vi "ManualLauncher.vi"() -> ()   [LabVIEW 2012]
uses:
  LauncherPresets.ctl
  Sally_Dashboard_2013/DBNameEnum.ctl
  Robot Global Data.vi
panel:
  in  "LauncherPresets":T1
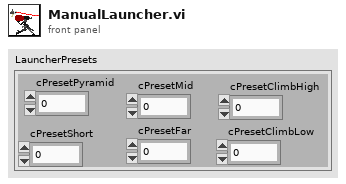
[diagram p1: front panel]
types:
  T1 = typedef "LauncherPresets.ctl" = cluster{"cPresetPyramid":dbl, "cPresetShort":dbl, "cPresetMid":dbl, "cPresetFar":dbl, "cPresetClimbHigh":dbl, "cPresetClimbLow":dbl}
  T2 = typedef "DBNameEnum.ctl" = enum16{"AutoInstructions", "DriveLoopTime", "DriveAlignLSLeft", "DriveAlignLSRight", "Use2DriveAlign", "ClimbLS", "LauncherAngleMatches", "FrameworkVersion", "sLauncherAngle", "LauncherTargetAngle", "sLauncherRPM", "LauncherTargetRPM", "sDriveDistance", "LauncherMotorValue", "PullbackTol", "FireTol", "LauncherRPMTol", "LauncherAngleTol", "InitialWait", "WaitBetweenLaunch", "AnglePresets", "RPMPresets", "UseAngleEncoder", "UseLauncherEncoder", "UseLauncherPID", "QSWaitBeforeFire", "QSWaitBeforeRetract", "AngleForwardValue", "AngleBackwardValue", "UseClusterArray", "BackupAuto", "ReverseDriveIndicate", "HalfSpeedFactor"}
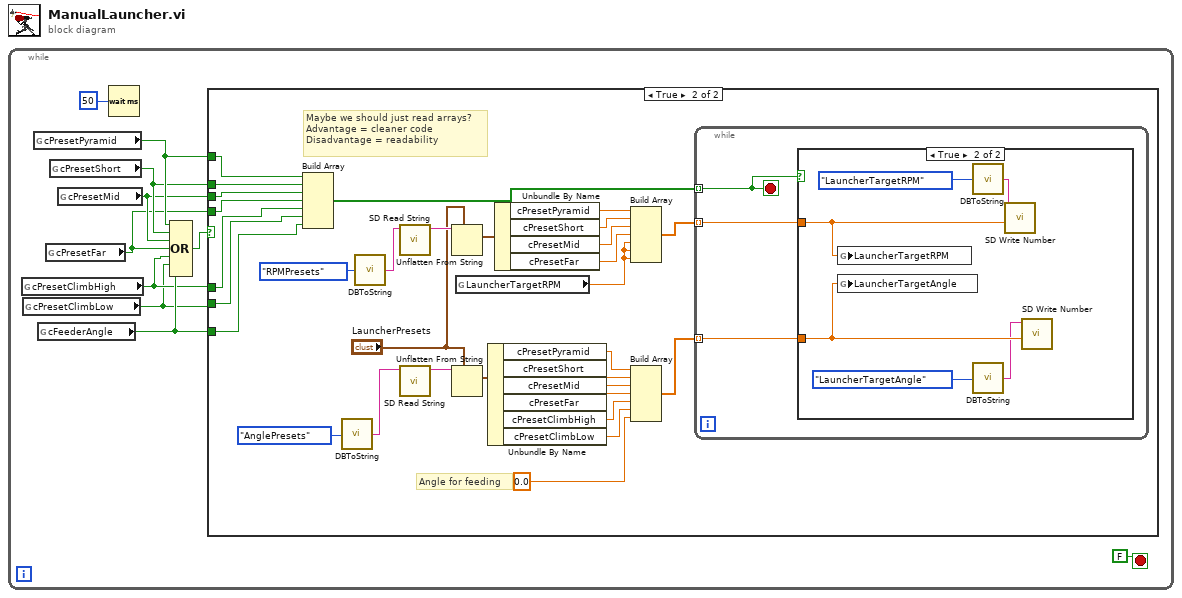
[diagram p0: block diagram]
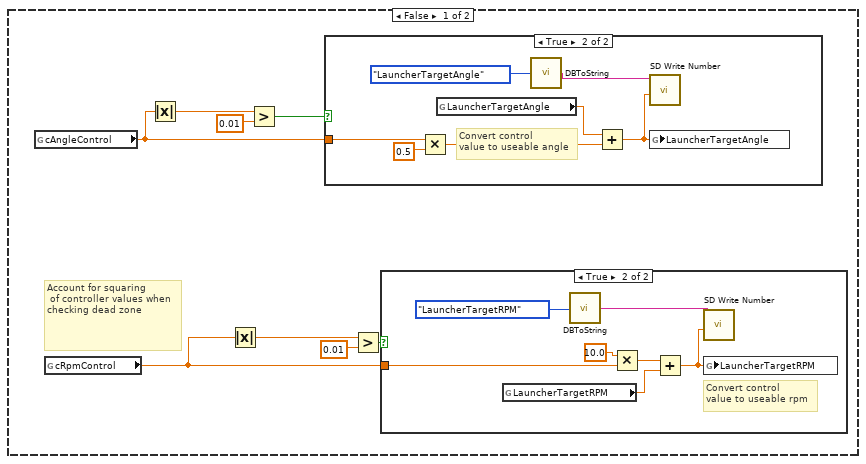
[diagram p2: hidden frame]
diagram:
  n1 = while {
    stop <- FALSE stop-if-true
    n2 = global read "Robot Global Data.vi" "cPresetClimbHigh"() -> (w2:bool)
    n3 = global read "Robot Global Data.vi" "cPresetClimbLow"() -> (w1:bool)
    n4 = global read "Robot Global Data.vi" "cPresetPyramid"() -> (w8:bool)
    n5 = global read "Robot Global Data.vi" "cFeederAngle"() -> (w3:bool)
    n6 = global read "Robot Global Data.vi" "cPresetFar"() -> (w5:bool)
    n7 = global read "Robot Global Data.vi" "cPresetShort"() -> (w7:bool)
    n8 = global read "Robot Global Data.vi" "cPresetMid"() -> (w6:bool)
    n9 = Wait (ms)(milliseconds to wait=u32 50) -> ()  [unwired: 1 out]
    n10 = Compound Arithmetic op=OR(w8, w7, w6, w5, w2, w1, w3) -> (w9:bool)
    n11 = case shown="True" w9 {
      tunnel: w8 -> [_ w63]
      tunnel: w7 -> [_ w62]
      tunnel: w6 -> [_ w61]
      tunnel: w5 -> [_ w60]
      tunnel: w3 -> [_ w33]
      tunnel: w2 -> [_ w35]
      tunnel: w1 -> [_ w34]
      frame False {
        # "Account for squaring\n of controller values when checking dead zone"
        n12 = global read "Robot Global Data.vi" "cAngleControl"() -> (w14:dbl)
        n13 = global read "Robot Global Data.vi" "cRpmControl"() -> (w16:dbl)
        n14 = Absolute Value(x=w14) -> (abs(x)=w15:dbl)
        n15 = Absolute Value(x=w16) -> (abs(x)=w17:dbl)
        n16 = Greater?(x=w15, y=0.01) -> (0:w13:bool)
        n17 = case shown="True" w13 {
          tunnel: w14 -> [_ w25]
          frame False {
          }
          frame True {
            # "Convert control\nvalue to useable angle"
            n18 = Multiply(x=w25, y=0.5) -> (x*y=w22:dbl)
            n19 = global read "Robot Global Data.vi" "LauncherTargetAngle"() -> (w23:dbl)
            n20 = call "DBToString.vi"("Enum"=DBNameEnum."LauncherTargetAngle") -> ("Refname"=w19:string)
            n21 = Add(x=w23, y=w22) -> (x+y=w21:dbl)
            n22 = call <vilib>:"SD Write Number.vi"("Numeric"=w21, "Name"=w19) -> ()  [unwired: 8 in, 2 out]
            n23 = global write "Robot Global Data.vi" "LauncherTargetAngle"(w21) -> ()
          }
        }
        n24 = Greater?(x=w17, y=0.01) -> (0:w12:bool)
        n25 = case shown="True" w12 {
          tunnel: w16 -> [_ w31]
          frame False {
          }
          frame True {
            # "Convert control\nvalue to useable rpm"
            n26 = global read "Robot Global Data.vi" "LauncherTargetRPM"() -> (w30:dbl)
            n27 = call "DBToString.vi"("Enum"=DBNameEnum."LauncherTargetRPM") -> ("Refname"=w26:string)
            n28 = Multiply(x=10.0, y=w31) -> (x*y=w29:dbl)
            n29 = Add(x=w29, y=w30) -> (x+y=w28:dbl)
            n30 = call <vilib>:"SD Write Number.vi"("Numeric"=w28, "Name"=w26) -> ()  [unwired: 8 in, 2 out]
            n31 = global write "Robot Global Data.vi" "LauncherTargetRPM"(w28) -> ()
          }
        }
      }
      frame True {
        # "Angle for feeding"
        # "Maybe we should just read arrays?\nAdvantage = cleaner code\nDisadvantage = readability"
        n32 = Build Array(w63, w62, w61, w60, w35, w34, w33) -> (w59:bool[])
        n33 = call "DBToString.vi"("Enum"=DBNameEnum."AnglePresets") -> ("Refname"=w40:string)
        n34 = call "DBToString.vi"("Enum"=DBNameEnum."RPMPresets") -> ("Refname"=w42:string)
        n35 = call <vilib>:"SD Read String.vi"("Name"=w42) -> ("String"=w51:string)  [unwired: 8 in, 2 out]
        n36 = call <vilib>:"SD Read String.vi"("Name"=w40) -> ("String"=w58:string)  [unwired: 8 in, 2 out]
        n37 = Unflatten From String(type="LauncherPresets", binary string=w51) -> (value=w49:T1)  [unwired: 3 in, 2 out]
        n38 = Unflatten From String(type="LauncherPresets", binary string=w58) -> (value=w57:T1)  [unwired: 3 in, 2 out]
        n39 = global read "Robot Global Data.vi" "LauncherTargetRPM"() -> (w39:dbl)
        n40 = Unbundle By Name(w57) -> ("cPresetPyramid"=w56:dbl, "cPresetShort"=w55:dbl, "cPresetMid"=w54:dbl, "cPresetFar"=w53:dbl, "cPresetClimbHigh"=w37:dbl, "cPresetClimbLow"=w36:dbl)
        n41 = Unbundle By Name(w49) -> ("cPresetPyramid"=w48:dbl, "cPresetShort"=w47:dbl, "cPresetMid"=w46:dbl, "cPresetFar"=w45:dbl)
        n42 = Build Array(w48, w47, w46, w45, w39, w39, w39) -> (w44:dbl[])
        n43 = Build Array(w56, w55, w54, w53, w37, w36, 0.0 ("element")) -> (w52:dbl[])
        n44 = while {
          tunnel: w59 -> [w66] mode=indexing
          tunnel: w52 -> [w65] mode=indexing
          tunnel: w44 -> [w64] mode=indexing
          stop <- w66 stop-if-true
          n45 = case shown="True" w66 {
            tunnel: w65 -> [_ w71]
            tunnel: w64 -> [_ w72]
            frame False {
            }
            frame True {
              n46 = global write "Robot Global Data.vi" "LauncherTargetRPM"(w72) -> ()
              n47 = global write "Robot Global Data.vi" "LauncherTargetAngle"(w71) -> ()
              n48 = call "DBToString.vi"("Enum"=DBNameEnum."LauncherTargetRPM") -> ("Refname"=w69:string)
              n49 = call "DBToString.vi"("Enum"=DBNameEnum."LauncherTargetAngle") -> ("Refname"=w68:string)
              n50 = call <vilib>:"SD Write Number.vi"("Numeric"=w72, "Name"=w69) -> ()  [unwired: 8 in, 2 out]
              n51 = call <vilib>:"SD Write Number.vi"("Numeric"=w71, "Name"=w68) -> ()  [unwired: 8 in, 2 out]
            }
          }
        }
      }
    }
  }
